vi "Start VI.vi"   [LabVIEW 2019]
types:
  T1 = typedef "队列枚举.ctl" = enum16{"ini", "读", "写"}
  T2 = enum16{"ini", "增", "删", "查", "改-通讯状态", "改-记录上限", "增-报文", "清空报文记录", "清空全部记录"}
  T3 = typedef "串口枚举.ctl" = enum16{"ini", "增", "删", "查", "改"}
  T4 = enum32{"Invalid", "Standard", "Closed", "Hidden", "Minimized", "Maximized"}
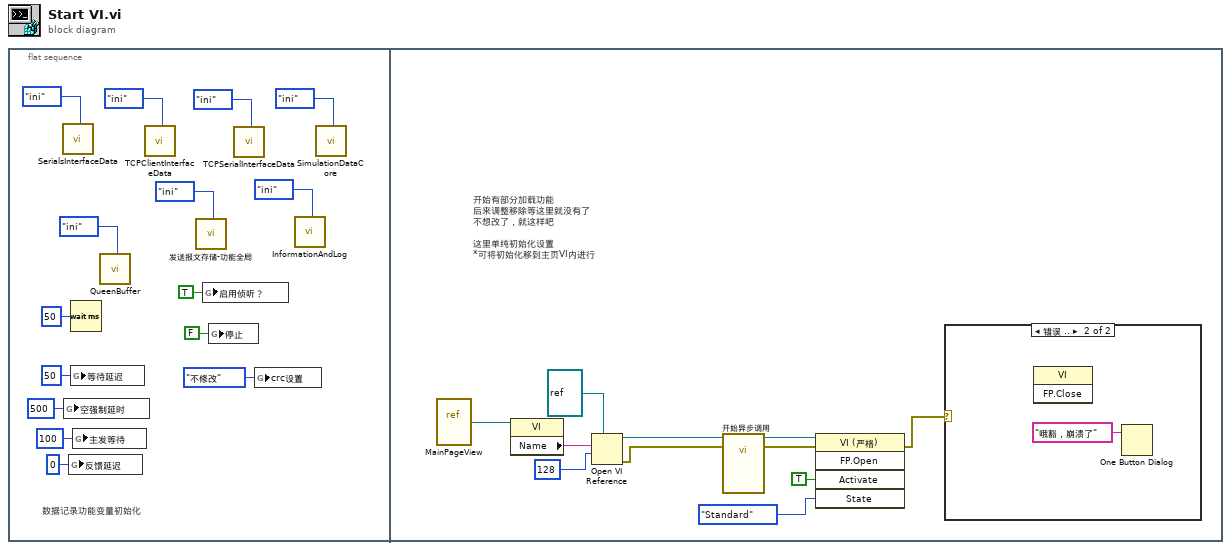
[diagram p0: block diagram]
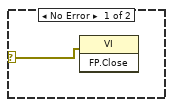
[diagram p2: hidden frame]
diagram:
  n1 = flat-sequence {
    frame #0 {
      # "数据记录功能变量初始化"
      n2 = call "SerialsInterfaceData.vi"("串口枚举"=串口枚举."ini") -> ()  [unwired: 17 in, 2 out]
      n3 = global write "全局-配置识别.vi" "空强制延时"(u32 500 ("空强制延时")) -> ()
      n4 = global write "全局-配置识别.vi" "反馈延迟"(u32 0 ("反馈延迟")) -> ()
      n5 = Wait (ms)(milliseconds to wait=u32 50 ("等待时间（毫秒）")) -> ()  [unwired: 1 out]
      n6 = global write "全局-配置识别.vi" "等待延迟"(u32 50 ("等待延迟")) -> ()
      n7 = global write "全局-配置识别.vi" "主发等待"(u32 100 ("主发等待")) -> ()
      n8 = call "QueenBuffer.vi"("操作"=队列枚举."ini") -> ()  [unwired: 18 in, 1 out]
      n9 = call "TCPClientInterfaceData.vi"("客服接口枚举"=enum16{"ini", "增", "删", "查", "改"}."ini") -> ()  [unwired: 17 in, 2 out]
      n10 = call "发送报文存储-功能全局.vi"("枚举"=enum16{"ini", "读", "写"}."ini") -> ()  [unwired: 18 in, 1 out]
      n11 = global write "全局-被反馈配置.vi" "启用侦听？"(TRUE ("启用反馈？")) -> ()
      n12 = global write "全局-配置识别.vi" "停止"(FALSE ("停止")) -> ()
      n13 = call "TCPSerialInterfaceData.vi"("客服接口枚举"=enum16{"ini", "增", "删", "查", "改", "腾笼换鸟"}."ini") -> ()  [unwired: 17 in, 2 out]
      n14 = global write "全局-被反馈配置.vi" "crc设置"(enum32{"不修改", "无CRC", "设置CRC"}."不修改" ("crc设置")) -> ()
      n15 = call "InformationAndLog.vi"("模拟数据枚举"=T2."ini") -> ()  [unwired: 17 in, 2 out]
      n16 = call "SimulationDataCore.vi"("模拟数据枚举"=enum16{"ini", "增", "删", "查", "改-全", "改-部分"}."ini") -> ()  [unwired: 17 in, 2 out]
    }
    frame #1 {
      # "开始有部分加载功能\n后来调整移除等这里就没有了\n不想改了，就这样吧\n\n这里单纯初始化设置\n*可将初始化移到主页VI内进行"
      n17 = vi-ref "MainPageView.vi"() -> (w22:refnum<vi>)
      n18 = property class="VI"(reference=w22) -> ("Name"=w26:string)  [unwired: 1 in, 2 out]
      n19 = Open VI Reference(type specifier VI Refnum (for type only)=refnum<vi> refnum ("类型说明符VI引用句柄（仅用于类型）"), vi path=w26, options=128 ("选项")) -> (vi reference=w25:refnum<vi>, error out=w16:errorcluster)  [unwired: 3 in]
      n20 = call-by-ref "开始异步调用"(reference=w25, error in=w16) -> (reference out=w21:refnum<vi>, error out=w20:errorcluster)  [unwired: 20 in]
      n21 = invoke class="VI (严格)" method="FP.Open"(reference=w21, error in=w20, "Activate"=TRUE ("激活？"), "State"=T4."Standard" ("状态")) -> (error out=w17:errorcluster)  [unwired: 1 in, 4 out]
      n22 = case shown="错误 .." w17 {
        selector: w17 -> [w27 _]
        frame No Error {
          n23 = invoke class="VI" method="FP.Close"(error in=w27) -> ()  [unwired: 2 in, 3 out]
        }
        frame Error {
          n24 = invoke class="VI" method="FP.Close"() -> ()  [unwired: 3 in, 3 out]
          n25 = One Button Dialog(message="哦豁，崩溃了" ("消息")) -> ()  [unwired: 1 in, 1 out]
        }
      }
    }
  }
